vi "GENser Formulate VI Call Chain.vi"(10 "Call Chain":string[](array[string])) -> (2 "String Out":string)   [LabVIEW 2017]
doc: "This VI accepts the caller VI's \"Call Chain\", which is an array of strings. It converts the string array into a string with \" -> \" between each element of the chain."
panel:
  # "Formulate VI Call Chain"
  # "Lambda Genesys \n Serial Port\n  DC Power Supplies"
  # "Create string that shows\nthe hierarchy of VI sub-calls"
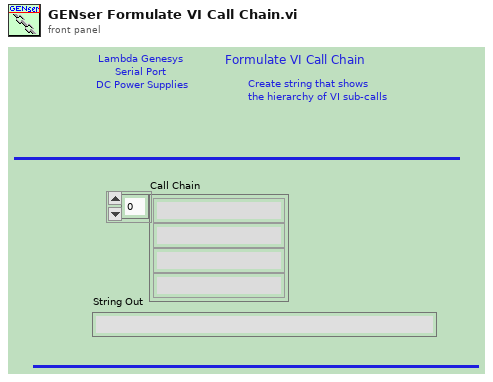
[diagram p1: front panel]
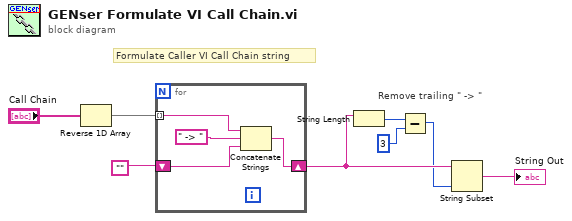
[diagram p0: block diagram]
diagram:
  # "Remove trailing \" -> \""
  # "Formulate Caller VI Call Chain string"
  n1 = Reverse 1D Array(array="Call Chain") -> (reversed array=w1:string[])
  n2 = for {
    tunnel: w1 -> [w12] mode=indexing
    shift-right: [w10] -> w5
    shift-left: "" -> [w9]
    n3 = Concatenate Strings(w12, " -> ", w9) -> (w10:string)
  }
  n4 = String Length(string=w5) -> (length=w7:i32)
  n5 = Subtract(x=w7, y=3) -> (x-y=w4:i32)
  n6 = String Subset(string=w5, length (rest)=w4) -> (substring=→"String Out":string)  [unwired: 1 in]
